vi "CRC_RSD.vi"(0 "BYTE 0":u16 format="%x", 1 "BYTE 1":u16 format="%x", 2 "BYTE 2":u16 format="%x", 3 "BYTE 3":u16 format="%x", 4 "Number of BYTE":u16) -> (5 "RSD":u16 format="%x")   [LabVIEW 2015]
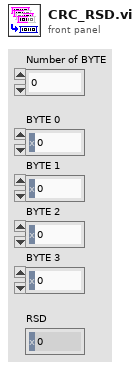
[diagram p1: front panel]
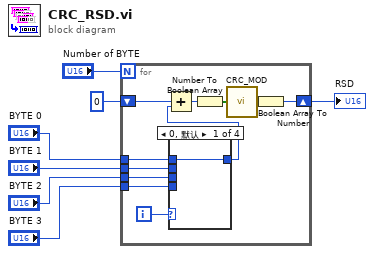
[diagram p0: block diagram]
diagram:
  n1 = for {
    N: "Number of BYTE" -> [_]
    shift-right: [w16] -> w2
    shift-left: 0 -> [w8]
    tunnel: "BYTE 0" -> [w13]
    tunnel: "BYTE 1" -> [w11]
    tunnel: "BYTE 2" -> [w10]
    tunnel: "BYTE 3" -> [w9]
    i -> [w14]
    n2 = case shown="0, 默认" w14 {
      tunnel: w13 -> [w19 _ _ _]
      tunnel: [w19 w20 w21 w22] -> w12
      tunnel: w11 -> [_ _ _ w22]
      tunnel: w10 -> [_ _ w21 _]
      tunnel: w9 -> [_ w20 _ _]
      frame 0, Default {
      }
      frame 3 {
      }
      frame 2 {
      }
      frame 1 {
      }
    }
    n3 = Add(x=w8, y=w12) -> (x+y=w15:u32)
    n4 = Number To Boolean Array(number=w15) -> (Boolean array=w18:bool[])
    n5 = call "CRC_MOD.vi"("输入"=w18) -> ("输出"=w17:bool[])
    n6 = Boolean Array To Number(Boolean array=w17) -> (number=w16:u32)
  }
  "RSD" <- w2
